vi "HFRR ADV v017 new software.vi"() -> ()   [LabVIEW 2025] (continued)
        n907 = call "IMAGE ANALYSIS.vi"("Enum"=POST_ANALYSIS_ENUM."SHOW UI", "error in"=w1071) -> ("error out"=w1069:errorcluster)  [unwired: 8 in, 1 out]
        n908 = local write "Zoom Factore"(100.0 ("Zoom Factore")) -> ()
      }
    }
    n909 = case shown="True" w760 {
      selector: w760 -> [_ w1048]
      tunnel: w752 -> [w1045 w1053]
      tunnel: [w1045 w1047] -> _
      frame False {
      }
      frame True {
        n910 = Not(x=w1048) -> (.not. x?=w1046:bool)
        n911 = local read "Zoom Factore"() -> (w1051:dbl)
        n912 = local write "OUT"(w1046) -> ()
        n913 = call "IMAGE ANALYSIS.vi"("Enum"=POST_ANALYSIS_ENUM."ZOOM OUT", "error in"=w1053) -> ("error out"=w1047:errorcluster)  [unwired: 8 in, 1 out]
        n914 = Divide(x=w1051, y=1.2) -> (x/y=w1049:dbl)
        n915 = local write "Zoom Factore"(w1049) -> ()
      }
    }
    n916 = case shown="True" w761 {
      selector: w761 -> [_ w1057]
      tunnel: w752 -> [w1054 w1062]
      tunnel: [w1054 w1055] -> _
      frame False {
      }
      frame True {
        n917 = Not(x=w1057) -> (.not. x?=w1056:bool)
        n918 = local read "Zoom Factore"() -> (w1060:dbl)
        n919 = local write "In"(w1056) -> ()
        n920 = call "IMAGE ANALYSIS.vi"("Enum"=POST_ANALYSIS_ENUM."ZOOM IN", "error in"=w1062) -> ("error out"=w1055:errorcluster)  [unwired: 8 in, 1 out]
        n921 = Multiply(x=w1060, y=1.2) -> (x*y=w1058:dbl)
        n922 = local write "Zoom Factore"(w1058) -> ()
      }
    }
    n923 = case shown="True" w757 {
      selector: w757 -> [_ w1029]
      tunnel: w752 -> [w1027 w1031]
      tunnel: [w1027 w1030] -> _
      frame False {
      }
      frame True {
        n924 = Not(x=w1029) -> (.not. x?=w1028:bool)
        n925 = local write "Clear ROI Tool"(w1028) -> ()
        n926 = call "IMAGE ANALYSIS.vi"("Enum"=POST_ANALYSIS_ENUM."CLEAR ROI", "error in"=w1031) -> ("error out"=w1030:errorcluster)  [unwired: 8 in, 1 out]
      }
    }
    n927 = case shown="True" w759 {
      selector: w759 -> [_ w1041]
      tunnel: w752 -> [w1039 w1044]
      tunnel: [w1039 w1042] -> _
      frame False {
      }
      frame True {
        n928 = Not(x=w1041) -> (.not. x?=w1040:bool)
        n929 = local write "line tool"(w1040) -> ()
        n930 = call "IMAGE ANALYSIS.vi"("Enum"=POST_ANALYSIS_ENUM."DRAW LINE", "error in"=w1044) -> ("error out"=w1042:errorcluster)  [unwired: 8 in, 1 out]
      }
    }
    n931 = case shown="True" w758 {
      selector: w758 -> [_ w1035]
      tunnel: w752 -> [w1033 w1037]
      tunnel: [w1033 w1036] -> _
      frame False {
      }
      frame True {
        n932 = Not(x=w1035) -> (.not. x?=w1034:bool)
        n933 = local write "Rectangle Tool"(w1034) -> ()
        n934 = call "IMAGE ANALYSIS.vi"("Enum"=POST_ANALYSIS_ENUM."DRAW REC", "error in"=w1037) -> ("error out"=w1036:errorcluster)  [unwired: 8 in, 1 out]
      }
    }
    n935 = local read "SCAR MEASURMENT"() -> (w745:enum32{"Auto Scar", "Manual Scar"})
    n936 = local read "Fit to Screen Tool"() -> (w754:bool)
    n937 = local read "Resize Tool"() -> (w753:bool)
    n938 = case shown="\"Manual Scar\", Default" w745 {
      frame "Auto Scar" {
        n939 = property on="Cap Live Image" class="Bool (strict)"("BoolText.Text"="Report" ("Boolean Text.Text")) -> ()  [unwired: 2 in, 2 out]
      }
      frame "Manual Scar", Default {
        n940 = property on="Cap Live Image" class="Bool (strict)"("BoolText.Text"="Save Image" ("Boolean Text.Text")) -> ()  [unwired: 2 in, 2 out]
      }
    }
    n941 = local read "ROI Color Tool"() -> (w755:bool)
    n942 = local read "Pan Tool"() -> (w756:bool)
    n943 = case shown="True" w756 {
      selector: w756 -> [_ w1023]
      tunnel: w752 -> [w1021 w1025]
      tunnel: [w1021 w1024] -> _
      frame False {
      }
      frame True {
        n944 = Not(x=w1023) -> (.not. x?=w1022:bool)
        n945 = call "IMAGE ANALYSIS.vi"("Enum"=POST_ANALYSIS_ENUM."PAN", "error in"=w1025) -> ("error out"=w1024:errorcluster)  [unwired: 8 in, 1 out]
        n946 = local write "Pan Tool"(w1022) -> ()
      }
    }
    n947 = case shown="True" w753 {
      selector: w753 -> [_ w1007]
      tunnel: w752 -> [w1002 w1004]
      tunnel: [w1002 w1003] -> _
      frame False {
      }
      frame True {
        n948 = Not(x=w1007) -> (.not. x?=w1006:bool)
        n949 = local write "Resize Tool"(w1006) -> ()
        n950 = call "IMAGE ANALYSIS.vi"("Enum"=POST_ANALYSIS_ENUM."RESIZE MODE", "error in"=w1004) -> ("error out"=w1003:errorcluster)  [unwired: 8 in, 1 out]
      }
    }
    n951 = case shown="True" w754 {
      selector: w754 -> [_ w1012]
      tunnel: [w1008 w1013] -> _
      tunnel: w752 -> [w1008 w1011]
      frame False {
      }
      frame True {
        n952 = Not(x=w1012) -> (.not. x?=w1010:bool)
        n953 = local write "Zoom Factore"(100.0 ("Zoom Factore")) -> ()
        n954 = local write "Fit to Screen Tool"(w1010) -> ()
        n955 = call "IMAGE ANALYSIS.vi"("Enum"=POST_ANALYSIS_ENUM."FIT", "error in"=w1011) -> ("error out"=w1013:errorcluster)  [unwired: 8 in, 1 out]
      }
    }
    n956 = case shown="True" w755 {
      selector: w755 -> [_ w1018]
      tunnel: [w1015 w1019] -> _
      tunnel: w752 -> [w1015 w1016]
      frame False {
      }
      frame True {
        n957 = Not(x=w1018) -> (.not. x?=w1017:bool)
        n958 = local write "ROI Color Tool"(w1017) -> ()
        n959 = call "IMAGE ANALYSIS.vi"("Enum"=POST_ANALYSIS_ENUM."SET ROI COLOR", "error in"=w1016) -> ("error out"=w1019:errorcluster)  [unwired: 8 in, 1 out]
      }
    }
    n960 = local read "Quit"() -> (w769:bool)
  }
  n961 = while {
    stop <- w1103 stop-if-true
    n962 = local read "Image Path"() -> (w1106:path)
    n963 = local read "Print 3"() -> (w1109:bool)
    n964 = Equal?(x=w1106, y=path "") -> (x = y?=w1105:bool)
    n965 = Not(x=w1105) -> (.not. x?=w1104:bool)
    n966 = property on="Print 3" class="Bool (strict)"("Visible"=w1104) -> ()  [unwired: 2 in, 2 out]
    n967 = case shown="True" w1109 {
      frame False {
        n968 = local write "Rd"(TRUE ("Boolean 7")) -> ()
      }
      frame True {
        n969 = flat-sequence {
          tunnel: [w1149] -> w1117
          tunnel: [w1136] -> w1115
          tunnel: [w1146] -> w1111
          tunnel: w1117 -> [w1158]
          tunnel: [w1158] -> w1116
          tunnel: w1115 -> [w1157]
          tunnel: [w1157] -> w1114
          tunnel: [w1155] -> w1113
          tunnel: [w1154] -> w1112
          tunnel: w1111 -> [w1154]
          tunnel: w1116 -> [w1160]
          tunnel: w1114 -> [w1161]
          tunnel: w1113 -> [_]
          tunnel: w1112 -> [w1159]
          frame #0 {
            n970 = case shown="True" "Rd" {
              frame False {
              }
              frame True {
                n971 = while {
                  tunnel: "abcdefABCDEF" ("string 2") -> [w1128]
                  shift-right: [w1126] -> w1120
                  shift-left: "" -> [w1125]
                  i -> [w1135]
                  stop <- w1134 stop-if-true
                  n972 = Random Number (0-1)() -> (number: 0 to 1=w1129:dbl)
                  n973 = Multiply(x=w1129, y=62.0) -> (x*y=w1131:dbl)
                  n974 = Decrement(x="Length 2") -> (x-1=w1124:i16)
                  n975 = To Word Integer(number=w1131) -> (16bit integer=w1132:i16)
                  n976 = String Subset(string=w1128, offset (0)=w1132, length (rest)=1 ("length (rest)")) -> (substring=w1127:string)
                  n977 = Greater Or Equal?(x=w1135, y=w1124) -> (x >= y?=w1134:bool)
                  n978 = Concatenate Strings(w1127, w1125) -> (w1126:string)
                }
                "String 10" <- w1120
                n979 = local write "Rd"(FALSE ("Boolean 7")) -> ()
              }
            }
          }
          frame #1 {
            w1147 = "_resized.jpg" ("command line")
            (unwired) ".jpg -resize 320x240 " ("string")
            (unwired) "Choose an Image File" ("prompt")
            # "-resize 1798x425"
            n980 = local read "Image Path"() -> (w1141:path)
            n981 = Strip Path(path=w1141) -> (stripped path=w1136:path, name=w1137:string)
            n982 = Match Pattern(string=w1137, regular expression=".jpg") -> (before substring=→"before substring 2":string, after substring=→"after substring":string)  [unwired: 1 in, 2 out]
            n983 = Match Pattern(string=w1137, regular expression="\\") -> (before substring=w1143:string)  [unwired: 1 in, 3 out]
            n984 = Match Pattern(string=w1143, regular expression=".jpg") -> (before substring=w1142:string)  [unwired: 1 in, 3 out]
            n985 = Concatenate Strings("cmd /c convert " ("string"), w1142, ".jpg -resize 320x240  " ("command line"), w1142, w1147) -> (w1150:string)
            n986 = call <vilib>:"System Exec.vi"("run minimized? (F)"=TRUE, "wait until completion? (T)"=TRUE, "working directory"=w1136, "command line"=w1150) -> ("error out"=w1149:errorcluster)  [unwired: 4 in, 3 out]
            "error out 2" <- w1149
            n987 = Concatenate Strings(w1142, w1147) -> (w1146:string)
          }
          frame #2 {
            n988 = Wait (ms)(milliseconds to wait=u32 2000 ("millisecond timer value")) -> (millisecond timer value=w1155:u32)
          }
          frame #3 {
            n989 = case shown="No Error" w1160 {
              tunnel: w1161 -> [w1164 _]
              tunnel: w1159 -> [w1162 _]
              frame No Error {
                (unwired) ".jpg" ("string")
                n990 = Path To String(path=w1164) -> (string=w1168:string)
                n991 = Concatenate Strings(w1168, "\\" ("string"), w1162) -> (w1167:string)
                n992 = String To Path(string=w1167) -> (path=w1166:path)
                n993 = call <vilib>:"Read JPEG File.vi"("path to JPEG file"=w1166) -> ("image data"=w1170:T16)  [unwired: 8 in, 2 out]
                "image data" <- w1170
                n994 = local write "Print 3"(FALSE ("Print 2")) -> ()
                n995 = call <vilib>:"Draw Flattened Pixmap.vi"("image data"=w1170) -> ("new picture"=→"new picture":picture)  [unwired: 8 in]
              }
              frame Error {
              }
            }
          }
        }
      }
    }
    n996 = Wait (ms)(milliseconds to wait=u32 20 ("millisecond timer value")) -> ()  [unwired: 1 out]
    n997 = local read "Quit"() -> (w1103:bool)
  }
  n998 = while {
    tunnel: w34 -> [_]
    tunnel: w18 -> [_]
    stop <- w1201 stop-if-true
    # "New Adv Logics"
    n999 = local read "Main Tab"() -> (w1181:T2)
    n1000 = local read "Main Tab"() -> (w1199:T2)
    n1001 = local read "Sign In"() -> (w1198:bool)
    n1002 = case shown="\"Adv Scar\"" w1181 {
      frame "HOME", Default {
        n1003 = local read "LIVE FEED MIN TEMP"() -> (w1334:bool)
        n1004 = local write "LIVE FEED MAX TEMP"(TRUE ("LIVE FEED MAX TEMP")) -> ()
        n1005 = local read "CAMERA ROI MIN TEMP"() -> (w1332:bool)
        n1006 = case shown="True" w1334 {
          selector: w1334 -> [_ w1341]
          frame False {
          }
          frame True {
            n1007 = Not(x=w1341) -> (.not. x?=w1340:bool)
            n1008 = local write "LIVE FEED MIN TEMP"(w1340) -> ()
            n1009 = call "CAMERA LIVE FEED FGV.vi"("Enum - Menu"=CAMERA_LIVE_FEED_ENUM."CAMERA MINIMIZE") -> ()  [unwired: 9 in, 2 out]
          }
        }
        n1010 = case shown="True" w1332 {
          selector: w1332 -> [_ w1338]
          frame False {
          }
          frame True {
            n1011 = Not(x=w1338) -> (.not. x?=w1337:bool)
            n1012 = local write "CAMERA ROI MIN TEMP"(w1337) -> ()
            n1013 = call "IMAGE ANALYSIS.vi"("Enum"=POST_ANALYSIS_ENUM."MINIMIZE UI") -> ()  [unwired: 9 in, 2 out]
          }
        }
        n1014 = local write "CAMERA ROI MAX TEMP"(TRUE ("CAMERA ROI MAX TEMP")) -> ()
      }
      frame "Test Setup" {
        n1015 = local read "LIVE FEED MIN TEMP"() -> (w1344:bool)
        n1016 = local read "CAMERA ROI MIN TEMP"() -> (w1342:bool)
        n1017 = local write "LIVE FEED MAX TEMP"(TRUE ("LIVE FEED MAX TEMP")) -> ()
        n1018 = case shown="True" w1344 {
          selector: w1344 -> [_ w1351]
          frame False {
          }
          frame True {
            n1019 = Not(x=w1351) -> (.not. x?=w1350:bool)
            n1020 = local write "LIVE FEED MIN TEMP"(w1350) -> ()
            n1021 = call "CAMERA LIVE FEED FGV.vi"("Enum - Menu"=CAMERA_LIVE_FEED_ENUM."CAMERA MINIMIZE") -> ()  [unwired: 9 in, 2 out]
          }
        }
        n1022 = case shown="True" w1342 {
          selector: w1342 -> [_ w1348]
          frame False {
          }
          frame True {
            n1023 = Not(x=w1348) -> (.not. x?=w1347:bool)
            n1024 = local write "CAMERA ROI MIN TEMP"(w1347) -> ()
            n1025 = call "IMAGE ANALYSIS.vi"("Enum"=POST_ANALYSIS_ENUM."MINIMIZE UI") -> ()  [unwired: 9 in, 2 out]
          }
        }
        n1026 = local write "CAMERA ROI MAX TEMP"(TRUE ("CAMERA ROI MAX TEMP")) -> ()
      }
      frame "Acquire" {
        n1027 = local read "LIVE FEED MIN TEMP"() -> (w1354:bool)
        n1028 = local write "LIVE FEED MAX TEMP"(TRUE ("LIVE FEED MAX TEMP")) -> ()
        n1029 = local read "CAMERA ROI MIN TEMP"() -> (w1352:bool)
        n1030 = case shown="True" w1354 {
          selector: w1354 -> [_ w1361]
          frame False {
          }
          frame True {
            n1031 = Not(x=w1361) -> (.not. x?=w1360:bool)
            n1032 = local write "LIVE FEED MIN TEMP"(w1360) -> ()
            n1033 = call "CAMERA LIVE FEED FGV.vi"("Enum - Menu"=CAMERA_LIVE_FEED_ENUM."CAMERA MINIMIZE") -> ()  [unwired: 9 in, 2 out]
          }
        }
        n1034 = case shown="True" w1352 {
          selector: w1352 -> [_ w1358]
          frame False {
          }
          frame True {
            n1035 = Not(x=w1358) -> (.not. x?=w1357:bool)
            n1036 = local write "CAMERA ROI MIN TEMP"(w1357) -> ()
            n1037 = call "IMAGE ANALYSIS.vi"("Enum"=POST_ANALYSIS_ENUM."MINIMIZE UI") -> ()  [unwired: 9 in, 2 out]
          }
        }
        n1038 = local write "CAMERA ROI MAX TEMP"(TRUE ("CAMERA ROI MAX TEMP")) -> ()
      }
      frame "Adv Scar" {
        n1039 = local read "CAMERA ROI MIN TEMP"() -> (w1362:bool)
        n1040 = case shown="True" "LIVE FEED MAX TEMP" {
          selector: "LIVE FEED MAX TEMP" -> [_ w1383]
          frame False {
          }
          frame True {
            n1041 = Not(x=w1383) -> (.not. x?=w1382:bool)
            n1042 = local write "LIVE FEED MAX TEMP"(w1382) -> ()
            n1043 = call "CAMERA LIVE FEED FGV.vi"("Enum - Menu"=CAMERA_LIVE_FEED_ENUM."CAMERA RESTORE") -> ("error out"=w1373:errorcluster)  [unwired: 9 in, 1 out]
            n1044 = Type Cast(type=30, x=0) -> (*(type *) &x=w1377:i32)
            n1045 = Add(x=w1377, y=48) -> (x+y=w1378:i32)
            n1046 = call "CAMERA LIVE FEED FGV.vi"("Enum - Menu"=CAMERA_LIVE_FEED_ENUM."CAMERA MODE SET", "error in (no error)"=w1373, "CAMERA MODE"=w1378) -> ("error out"=w1370:errorcluster)  [unwired: 7 in, 1 out]
            n1047 = call "CAMERA LIVE FEED FGV.vi"("Enum - Menu"=CAMERA_LIVE_FEED_ENUM."CAMERA GRAY", "error in (no error)"=w1370) -> ("error out"=w1369:errorcluster)  [unwired: 8 in, 1 out]
            n1048 = call "LIST FILE NAMES.vi"("error in (no error)"=w1369) -> ("error out"=w1379:errorcluster, "filenames"=w1380:string[])  [unwired: 9 in]
            n1049 = property on="FILE 3" class="CmbBox"(error in=w1379, "Strings[]"=w1380) -> ()  [unwired: 1 in, 2 out]
          }
        }
        n1050 = case shown="True" w1362 {
          selector: w1362 -> [_ w1368]
          frame False {
          }
          frame True {
            n1051 = Not(x=w1368) -> (.not. x?=w1367:bool)
            n1052 = local write "CAMERA ROI MIN TEMP"(w1367) -> ()
            n1053 = call "IMAGE ANALYSIS.vi"("Enum"=POST_ANALYSIS_ENUM."MINIMIZE UI") -> ()  [unwired: 9 in, 2 out]
          }
        }
        n1054 = local write "CAMERA ROI MAX TEMP"(TRUE ("CAMERA ROI MAX TEMP")) -> ()
        "LIVE FEED MIN TEMP" <- TRUE ("LIVE FEED MIN TEMP")
      }
      frame "Adv Scar Report" {
        n1055 = local read "CAMERA ROI MAX TEMP"() -> (w1384:bool)
        n1056 = local read "LIVE FEED MIN TEMP"() -> (w1386:bool)
        n1057 = local write "LIVE FEED MAX TEMP"(TRUE ("LIVE FEED MAX TEMP")) -> ()
        n1058 = case shown="True" w1386 {
          selector: w1386 -> [_ w1395]
          frame False {
          }
          frame True {
            n1059 = Not(x=w1395) -> (.not. x?=w1394:bool)
            n1060 = local write "LIVE FEED MIN TEMP"(w1394) -> ()
            n1061 = call "CAMERA LIVE FEED FGV.vi"("Enum - Menu"=CAMERA_LIVE_FEED_ENUM."CAMERA MINIMIZE") -> ()  [unwired: 9 in, 2 out]
          }
        }
        n1062 = case shown="True" w1384 {
          selector: w1384 -> [_ w1392]
          frame False {
          }
          frame True {
            n1063 = Not(x=w1392) -> (.not. x?=w1390:bool)
            n1064 = local write "CAMERA ROI MAX TEMP"(w1390) -> ()
            n1065 = call "IMAGE ANALYSIS.vi"("Enum"=POST_ANALYSIS_ENUM."SHOW UI") -> ("error out"=w1389:errorcluster)  [unwired: 9 in, 1 out]
            n1066 = call "LIST FILE NAMES.vi"("error in (no error)"=w1389) -> ("filenames"=w1388:string[])  [unwired: 9 in, 1 out]
            n1067 = property on="Test File List :" class="CmbBox"("Strings[]"=w1388) -> ()  [unwired: 2 in, 2 out]
          }
        }
        n1068 = local write "CAMERA ROI MIN TEMP"(TRUE ("CAMERA ROI MIN TEMP")) -> ()
      }
      frame "Compare Files" {
        n1069 = local read "LIVE FEED MIN TEMP"() -> (w1398:bool)
        n1070 = local write "LIVE FEED MAX TEMP"(TRUE ("LIVE FEED MAX TEMP")) -> ()
        n1071 = local read "CAMERA ROI MIN TEMP"() -> (w1396:bool)
        n1072 = case shown="True" w1398 {
          selector: w1398 -> [_ w1405]
          frame False {
          }
          frame True {
            n1073 = Not(x=w1405) -> (.not. x?=w1404:bool)
            n1074 = local write "LIVE FEED MIN TEMP"(w1404) -> ()
            n1075 = call "CAMERA LIVE FEED FGV.vi"("Enum - Menu"=CAMERA_LIVE_FEED_ENUM."CAMERA MINIMIZE") -> ()  [unwired: 9 in, 2 out]
          }
        }
        n1076 = case shown="True" w1396 {
          selector: w1396 -> [_ w1402]
          frame False {
          }
          frame True {
            n1077 = Not(x=w1402) -> (.not. x?=w1401:bool)
            n1078 = local write "CAMERA ROI MIN TEMP"(w1401) -> ()
            n1079 = call "IMAGE ANALYSIS.vi"("Enum"=POST_ANALYSIS_ENUM."MINIMIZE UI") -> ()  [unwired: 9 in, 2 out]
          }
        }
        n1080 = local write "CAMERA ROI MAX TEMP"(TRUE ("CAMERA ROI MAX TEMP")) -> ()
      }
      frame "About" {
        n1081 = local read "LIVE FEED MIN TEMP"() -> (w1408:bool)
        n1082 = local write "LIVE FEED MAX TEMP"(TRUE ("LIVE FEED MAX TEMP")) -> ()
        n1083 = local read "CAMERA ROI MIN TEMP"() -> (w1407:bool)
        n1084 = case shown="True" w1408 {
          selector: w1408 -> [_ w1415]
          frame False {
          }
          frame True {
            n1085 = Not(x=w1415) -> (.not. x?=w1414:bool)
            n1086 = local write "LIVE FEED MIN TEMP"(w1414) -> ()
            n1087 = call "CAMERA LIVE FEED FGV.vi"("Enum - Menu"=CAMERA_LIVE_FEED_ENUM."CAMERA MINIMIZE") -> ()  [unwired: 9 in, 2 out]
          }
        }
        n1088 = case shown="True" w1407 {
          selector: w1407 -> [_ w1412]
          frame False {
          }
          frame True {
            n1089 = Not(x=w1412) -> (.not. x?=w1411:bool)
            n1090 = local write "CAMERA ROI MIN TEMP"(w1411) -> ()
            n1091 = call "IMAGE ANALYSIS.vi"("Enum"=POST_ANALYSIS_ENUM."MINIMIZE UI") -> ()  [unwired: 9 in, 2 out]
          }
        }
        n1092 = local write "CAMERA ROI MAX TEMP"(TRUE ("CAMERA ROI MIN TEMP")) -> ()
      }
      frame "Advance" {
        n1093 = local read "LIVE FEED MIN TEMP"() -> (w1418:bool)
        n1094 = local write "LIVE FEED MAX TEMP"(TRUE ("LIVE FEED MAX TEMP")) -> ()
        n1095 = local read "CAMERA ROI MIN TEMP"() -> (w1416:bool)
        n1096 = case shown="True" w1418 {
          selector: w1418 -> [_ w1425]
          frame False {
          }
          frame True {
            n1097 = Not(x=w1425) -> (.not. x?=w1424:bool)
            n1098 = local write "LIVE FEED MIN TEMP"(w1424) -> ()
            n1099 = call "CAMERA LIVE FEED FGV.vi"("Enum - Menu"=CAMERA_LIVE_FEED_ENUM."CAMERA MINIMIZE") -> ()  [unwired: 9 in, 2 out]
          }
        }
        n1100 = local write "CAMERA ROI MAX TEMP"(TRUE ("CAMERA ROI MAX TEMP")) -> ()
        n1101 = case shown="True" w1416 {
          selector: w1416 -> [_ w1422]
          frame False {
          }
          frame True {
            n1102 = Not(x=w1422) -> (.not. x?=w1421:bool)
            n1103 = local write "CAMERA ROI MIN TEMP"(w1421) -> ()
            n1104 = call "IMAGE ANALYSIS.vi"("Enum"=POST_ANALYSIS_ENUM."MINIMIZE UI") -> ()  [unwired: 9 in, 2 out]
          }
        }
      }
      frame "Mooha" {
        n1105 = local read "LIVE FEED MIN TEMP"() -> (w1428:bool)
        n1106 = local write "LIVE FEED MAX TEMP"(TRUE ("LIVE FEED MAX TEMP")) -> ()
        n1107 = local read "CAMERA ROI MIN TEMP"() -> (w1426:bool)
        n1108 = case shown="True" w1428 {
          selector: w1428 -> [_ w1435]
          frame False {
          }
          frame True {
            n1109 = Not(x=w1435) -> (.not. x?=w1434:bool)
            n1110 = local write "LIVE FEED MIN TEMP"(w1434) -> ()
            n1111 = call "CAMERA LIVE FEED FGV.vi"("Enum - Menu"=CAMERA_LIVE_FEED_ENUM."CAMERA MINIMIZE") -> ()  [unwired: 9 in, 2 out]
          }
        }
        n1112 = local write "CAMERA ROI MAX TEMP"(TRUE ("CAMERA ROI MAX TEMP")) -> ()
        n1113 = case shown="True" w1426 {
          selector: w1426 -> [_ w1432]
          frame False {
          }
          frame True {
            n1114 = Not(x=w1432) -> (.not. x?=w1431:bool)
            n1115 = local write "CAMERA ROI MIN TEMP"(w1431) -> ()
            n1116 = call "IMAGE ANALYSIS.vi"("Enum"=POST_ANALYSIS_ENUM."MINIMIZE UI") -> ()  [unwired: 9 in, 2 out]
          }
        }
      }
    }
    n1117 = local read "Auto Start Test"() -> (w1172:bool)
    n1118 = case shown="True" "sign in temp" {
      frame False {
      }
      frame True {
        w1208 = 1 ("y")
        n1119 = local read "USERNAME"() -> (w1214:string)
        n1120 = local read "USER ID"() -> (w1211:string)
        n1121 = call <vilib>:"Trim Whitespace.vi"("string"=w1214) -> ("trimmed string"=w1213:string)  [unwired: 1 in]
        n1122 = call <vilib>:"Trim Whitespace.vi"("string"=w1211) -> ("trimmed string"=w1212:string)  [unwired: 1 in]
        n1123 = String Length(string=w1213) -> (length=w1210:i32)
        n1124 = String Length(string=w1212) -> (length=w1209:i32)
        n1125 = Greater?(x=w1210, y=w1208) -> (0:w1207:bool)
        n1126 = Greater?(x=w1209, y=w1208) -> (0:w1206:bool)
        n1127 = And(x=w1207, y=w1206) -> (x .and. y?=w1205:bool)
        n1128 = case shown="True" w1205 {
          frame False {
            n1129 = property on="Sign In" class="Bool (strict)"("DisabledEnum"=T19."Disabled" ("Disabled")) -> ()  [unwired: 2 in, 2 out]
          }
          frame True {
            n1130 = property on="Sign In" class="Bool (strict)"("DisabledEnum"=T19."Enabled" ("Disabled")) -> ()  [unwired: 2 in, 2 out]
          }
        }
      }
    }
    n1131 = local read "Air Temperature"() -> (w1189:bool)
    n1132 = local read "Coefficient Of Friction"() -> (w1190:bool)
    n1133 = case shown="False" w1172 {
      frame False {
        n1134 = local read "Auto stop temp"() -> (w1202:bool)
        n1135 = case shown="True" w1202 {
          frame False {
          }
          frame True {
            n1136 = local write "Auto Start Temp"(FALSE ("Auto Start Temp")) -> ()
          }
        }
      }
      frame True {
        "Auto stop temp" <- TRUE ("Auto stop temp")
      }
    }
    n1137 = local read "Humidity"() -> (w1188:bool)
    n1138 = case shown="\"HOME\"" w1199 {
      frame "HOME" {
        n1139 = local write "main tab sub"(enum32{"Page 1", "Page 2"}."Page 1" ("main tab sub")) -> ()
      }
      frame Default {
        n1140 = local write "main tab sub"(enum32{"Page 1", "Page 2"}."Page 2" ("main tab sub")) -> ()
      }
    }
    n1141 = case shown="True" w1198 {
      selector: w1198 -> [_ w1549]
      frame False {
      }
      frame True {
        n1142 = Not(x=w1549) -> (.not. x?=w1548:bool)
        n1143 = local write "Sign In"(w1548) -> ()
        n1144 = local write "Main Dashboard Buttons"(T24."Test Setup" ("Main Dashboard Buttons")) -> ()
      }
    }
    n1145 = case shown="\"Numeric Display\", Default" "Num/Graph" {
      frame "Numeric Display", Default {
        n1146 = property on="Single/Multiple" class="RadioBtnsControl (strict)"("Visible"=FALSE) -> ()  [unwired: 2 in, 2 out]
        n1147 = property on="Single - Graph" class="Ring (strict)"("Visible"=FALSE) -> ()  [unwired: 2 in, 2 out]
        n1148 = local write "Main Tab Display"(T4."Dashboard 1" ("Main Tab Display")) -> ()
      }
      frame "Graph Display" {
        n1149 = property on="Single/Multiple" class="RadioBtnsControl (strict)"("Visible"=TRUE) -> ()  [unwired: 2 in, 2 out]
        n1150 = case shown="\"Multiple\"" "Single/Multiple" {
          frame "Single ", Default {
            n1151 = property on="Single - Graph" class="Ring (strict)"("Visible"=TRUE) -> ()  [unwired: 2 in, 2 out]
            n1152 = local write "Main Tab Display"(T4."Dashboard 3" ("Main Tab Display")) -> ()
          }
          frame "Multiple" {
            n1153 = property on="Single - Graph" class="Ring (strict)"("Visible"=FALSE) -> ()  [unwired: 2 in, 2 out]
            n1154 = local write "Main Tab Display"(T4."Dashboard 2" ("Main Tab Display")) -> ()
          }
        }
      }
    }
    n1155 = local read "Stroke"() -> (w1187:bool)
    n1156 = local read "USERNAME"() -> (w1193:string)
    n1157 = local read "USER ID"() -> (w1192:string)
    n1158 = case shown="True" w1190 {
      selector: w1190 -> [_ w1475]
      frame False {
      }
      frame True {
        n1159 = Not(x=w1475) -> (.not. x?=w1474:bool)
        n1160 = local write "Coefficient Of Friction"(w1474) -> ()
        n1161 = local write "Tab Control 2"(T6."Coefficient Of Friction" ("Tab Control 2")) -> ()
      }
    }
    n1162 = case shown="True" w1189 {
      selector: w1189 -> [_ w1472]
      frame False {
      }
      frame True {
        n1163 = Not(x=w1472) -> (.not. x?=w1470:bool)
        n1164 = local write "Air Temperature"(w1470) -> ()
        n1165 = local write "Tab Control 2"(T6."Air Temperature" ("Tab Control 2")) -> ()
      }
    }
    n1166 = local write "Operator ID"(w1192) -> ()
    n1167 = case shown="True" w1187 {
      selector: w1187 -> [_ w1466]
      frame False {
      }
      frame True {
        n1168 = Not(x=w1466) -> (.not. x?=w1464:bool)
        n1169 = local write "Stroke"(w1464) -> ()
        n1170 = local write "Tab Control 2"(T6."Stroke" ("Tab Control 2")) -> ()
      }
    }
    n1171 = local write "tested by"(w1193) -> ()
    n1172 = case shown="True" w1188 {
      selector: w1188 -> [_ w1469]
      frame False {
      }
      frame True {
        n1173 = Not(x=w1469) -> (.not. x?=w1467:bool)
        n1174 = local write "Humidity"(w1467) -> ()
        n1175 = local write "Tab Control 2"(T6."Humidity" ("Tab Control 2")) -> ()
      }
    }
    n1176 = case shown="\"Calibration\"" "Main Dashboard Buttons" {
      tunnel: [T2."HOME" ("Main Tab") T2."Test Setup" ("Main Tab") T2."Acquire" ("Main Tab") T2."Adv Scar" ("Main Tab") T2."Adv Scar Report" ("Main Tab") T2."Compare Files" ("Main Tab") T2."Calibration" ("Main Tab") T2."About" ("Main Tab") T2."Advance" ("Main Tab")] -> w1171
      frame "Home", Default {
      }
      frame "Test Setup" {
      }
      frame "Dashboard" {
      }
      frame "Imaging" {
      }
      frame "Report" {
      }
      frame "Analysis" {
      }
      frame "Calibration" {
      }
      frame "About" {
      }
      frame "Advance" {
      }
    }
    n1177 = Wait (ms)(milliseconds to wait=u32 100) -> ()  [unwired: 1 out]
    n1178 = local read "Main Tab Display"() -> (w1191:T4)
    n1179 = local write "Main Tab"(w1171) -> ()
    n1180 = case shown="\"Dashboard 3\"" w1191 {
      frame "Dashboard 1", Default {
        n1181 = property on="Reset Graph" class="Bool (strict)"("Visible"=FALSE) -> ()  [unwired: 2 in, 2 out]
      }
      frame "Dashboard 2" {
        n1182 = property on="Reset Graph" class="Bool (strict)"("Visible"=TRUE) -> ()  [unwired: 2 in, 2 out]
      }
      frame "Dashboard 3" {
        n1183 = property on="Reset Graph" class="Bool (strict)"("Visible"=TRUE) -> ()  [unwired: 2 in, 2 out]
      }
    }
    n1184 = local read "SCAR MEASURMENT"() -> (w1179:enum32{"Auto Scar", "Manual Scar"})
    n1185 = local read "Humidity"() -> (w1194:bool)
    n1186 = local read "Cap Live Image"() -> (w1176:bool)
    n1187 = local read "Sample Temperature"() -> (w1186:bool)
    n1188 = local read "Air Temp vs Humidity"() -> (w1184:bool)
    n1189 = local read "Frequency"() -> (w1185:bool)
    n1190 = case shown="True" w1194 {
      frame False {
        n1191 = local write "Humidity On Command"(TRUE ("Humidity On Command")) -> ()
        n1192 = case shown="True" "Humidity Off Command" {
          selector: "Humidity Off Command" -> [_ w1482]
          frame False {
          }
          frame True {
            n1193 = stacked-sequence {
              frame #0 {
                n1194 = local read "WriteHumidity"() -> (w1484:string[])
                n1195 = Insert Into Array(array=w1484, new element="R;1" ("new element/subarray")) -> (w1485:string[])  [unwired: 1 in]
                n1196 = local write "WriteHumidity"(w1485) -> ()
              }
              frame #1 {
                n1197 = Wait (ms)(milliseconds to wait=u32 2000) -> ()  [unwired: 1 out]
              }
              frame #2 {
                n1198 = local read "EVENT LOG"() -> (w1491:string)
                n1199 = local read "WriteHumidity"() -> (w1488:string[])
                n1200 = call "Event Log.vi"("Content"="Humidity Control Off" ("string"), "EVENT LOG"=w1491) -> ("EVENT LOG"=w1492:string)  [unwired: 8 in, 1 out]
                n1201 = local write "EVENT LOG"(w1492) -> ()
                n1202 = Insert Into Array(array=w1488, new element="R;1" ("new element/subarray")) -> (w1489:string[])  [unwired: 1 in]
                n1203 = local write "WriteHumidity"(w1489) -> ()
              }
            }
            n1204 = Not(x=w1482) -> (.not. x?=w1481:bool)
            n1205 = local write "Humidity Off Command"(w1481) -> ()
          }
        }
      }
      frame True {
        n1206 = local write "Humidity Off Command"(TRUE ("Humidity Off Command")) -> ()
        n1207 = case shown="True" "Humidity On Command" {
          selector: "Humidity On Command" -> [_ w1496]
          frame False {
          }
          frame True {
            n1208 = stacked-sequence {
              frame #0 {
                n1209 = local read "Set Rh"() -> (w1502:dbl)
                n1210 = Number To Fractional String(number=w1502, precision (6)=i16 2) -> (F-format string=w1503:string)  [unwired: 2 in]
                n1211 = local read "WriteHumidity"() -> (w1500:string[])
                n1212 = Concatenate Strings("M;" ("new element/subarray"), w1503) -> (w1501:string)
                n1213 = Insert Into Array(array=w1500, new element=w1501) -> (w1499:string[])  [unwired: 1 in]
                n1214 = local write "WriteHumidity"(w1499) -> ()
              }
              frame #1 {
                n1215 = Wait (ms)(milliseconds to wait=u32 2000) -> ()  [unwired: 1 out]
              }
              frame #2 {
                n1216 = local read "Set Rh"() -> (w1510:dbl)
                n1217 = Number To Fractional String(number=w1510, precision (6)=i16 2) -> (F-format string=w1511:string)  [unwired: 2 in]
                n1218 = local read "WriteHumidity"() -> (w1508:string[])
                n1219 = Concatenate Strings("M;" ("new element/subarray"), w1511) -> (w1509:string)
                n1220 = Insert Into Array(array=w1508, new element=w1509) -> (w1507:string[])  [unwired: 1 in]
                n1221 = local write "WriteHumidity"(w1507) -> ()
              }
              frame #3 {
                n1222 = Wait (ms)(milliseconds to wait=u32 1500) -> ()  [unwired: 1 out]
              }
              frame #4 {
                (unwired) "% RH" ("string")
                (unwired) i16 2 ("precision (6)")
                (unwired) "M;" ("new element/subarray")
                n1223 = local read "Set Rh"() -> (w1518:dbl)
                n1224 = Number To Fractional String(number=w1518, precision (6)=i16 2) -> (F-format string=w1515:string)  [unwired: 2 in]
                n1225 = local read "WriteHumidity"() -> (w1520:string[])
                n1226 = Concatenate Strings("M;" ("new element/subarray"), w1515) -> (w1519:string)
                n1227 = Concatenate Strings("Humidity Set to : " ("string"), w1515, "% RH" ("string")) -> (w1513:string)
                n1228 = Insert Into Array(array=w1520, new element=w1519) -> (w1521:string[])  [unwired: 1 in]
                n1229 = disable-structure shown="Enabled" {
                  frame Enabled {
                    n1230 = local read "EVENT LOG"() -> (w1524:string)
                    n1231 = call "Event Log.vi"("Content"="Humidity Control On", "EVENT LOG"=w1524) -> ("EVENT LOG"=w1525:string)  [unwired: 8 in, 1 out]
                    n1232 = local write "EVENT LOG"(w1525) -> ()
                  }
                  frame Disabled {
                  }
                }
                n1233 = disable-structure shown="Enabled" {
                  disable-tunnel: w1513 -> [_ _]
                  frame Enabled {
                    n1234 = local read "EVENT LOG"() -> (w1527:string)
                    n1235 = call "Event Log.vi"("Content"="Humidity Control On", "EVENT LOG"=w1527) -> ("EVENT LOG"=w1528:string)  [unwired: 8 in, 1 out]
                    n1236 = local write "EVENT LOG"(w1528) -> ()
                  }
                  frame Disabled {
                  }
                }
                n1237 = local write "WriteHumidity"(w1521) -> ()
              }
            }
            n1238 = Not(x=w1496) -> (.not. x?=w1495:bool)
            n1239 = local write "Humidity On Command"(w1495) -> ()
          }
        }
      }
    }
    n1240 = Equal?(x=w1179, y=enum32{"Auto Scar", "Manual Scar"}."Auto Scar" ("SCAR MEASURMENT")) -> (x = y?=w1175:bool)
    n1241 = local read "TEST STANDARD"() -> (w1182:T3)
    n1242 = And(x=w1176, y=w1175) -> (x .and. y?=w1177:bool)
    n1243 = case shown="True" w1177 {
      selector: w1177 -> [_ w1281]
      tunnel: errorcluster {"status"=FALSE, "code"=0, "source"=""} ("error in (no error) 3") -> [_ w1282]
      frame False {
      }
      frame True {
        n1244 = stacked-sequence {
          tunnel: w1282 -> [_ _ _ _ _ _ _ w1330]
          tunnel: w1281 -> [_ _ _ _ _ w1311 _ _]
          frame #0 {
            n1245 = call "CAMERA LIVE FEED FGV.vi"("Enum - Menu"=CAMERA_LIVE_FEED_ENUM."CAMERA MINIMIZE") -> ()  [unwired: 9 in, 2 out]
          }
          frame #1 {
            n1246 = property on="Auto Scar Check  2" class="Clust (strict)"("Visible"=TRUE) -> ()  [unwired: 2 in, 2 out]
          }
          frame #2 {
            n1247 = String To Path(string="C:\\LAB-IQ\\Image Calibrate v01.dcf") -> (path=w1287:path)
            n1248 = Open/Create/Replace File ("Open File")(file path (use dialog)=w1287) -> (refnum out=w1288:refnum<file>)  [unwired: 5 in, 2 out]
            n1249 = for {
              N: 4 -> [_]
              tunnel: w1288 -> [w1294]
              i -> [w1290]
              n1250 = Read from Text File ("Read File")(file (use dialog)=w1294) -> (text=w1295:string)  [unwired: 3 in, 3 out]
              n1251 = String Subset(string=w1295, offset (0)=6, length (rest)=10 ("length (rest)")) -> (substring=w1291:string)
              n1252 = Fract/Exp String To Number(string=w1291) -> (number=w1289:dbl)  [unwired: 3 in, 1 out]
              n1253 = case shown="0" w1290 {
                tunnel: w1289 -> [w1296 w1297 _ w1298 _]
                frame 0 {
                  "5x Gain" <- w1296
                }
                frame 1 {
                  "10x Gain" <- w1297
                }
                frame 2 {
                }
                frame 3 {
                  "100x gain" <- w1298
                }
                frame 4, Default {
                }
              }
            }
          }
          frame #3 {
            n1254 = local read "FILE 3"() -> (w1304:string)
            n1255 = call <vilib>:"Trim Whitespace.vi"("string"="C:\\LAB-IQ\\images\\") -> ("trimmed string"=w1306:string)  [unwired: 1 in]
            n1256 = String To Path(string=w1306) -> (path=w1305:path)
            n1257 = Concatenate Strings(w1304, ".png" ("string")) -> (w1303:string)
            n1258 = Build Path(base path=w1305, name or relative path=w1303) -> (appended path=w1301:path)
            "Image path" <- w1301
            n1259 = Path To String(path=w1301) -> (string=w1300:string)
            n1260 = call "CAMERA LIVE FEED FGV.vi"("Enum - Menu"=CAMERA_LIVE_FEED_ENUM."CAMERA SAVE", "Image Path"=w1300) -> ()  [unwired: 8 in, 2 out]
          }
          frame #4 {
            n1261 = One Button Dialog(message="Image saved successfully") -> ()  [unwired: 1 in, 1 out]
          }
          frame #5 {
            n1262 = local read "TEST STANDARD"() -> (w1310:T3)
            n1263 = local read "Magnification len live scar"() -> (w1322:string)
            n1264 = Not(x=w1311) -> (.not. x?=w1312:bool)
            n1265 = local write "Cap Live Image"(w1312) -> ()
            n1266 = case shown="\"ISO 12156\"" w1310 {
              tunnel: ["ASTM D6079" "ISO 12156"] -> w1309
              frame "ASTM D6079", Default {
              }
              frame "ISO 12156" {
              }
            }
            n1267 = case shown="\"5x\", Default" w1322 {
              tunnel: [w1325 w1326] -> w1321
              frame "5x", Default {
                n1268 = local read "5x Gain"() -> (w1325:dbl)
              }
              frame "10x" {
                # "5x"
                n1269 = local read "10x Gain"() -> (w1326:dbl)
              }
            }
            n1270 = local read "Image path"() -> (w1320:path)
            n1271 = local read "FILE 3"() -> (w1313:string)
            n1272 = call "EDGE DETCTION.vi"("GAIN VALUE"=w1321, "Image Path"=w1320) -> ("error out"=w1319:errorcluster, "return value"=w1318:cluster{string, string, dbl, dbl, dbl})  [unwired: 8 in]
            n1273 = Bundle By Name(cluster=T25 {"File Name"="", "Test Method"="", "Operator"="", "Fuel Description"="", "Date and time"=""} ("Main Ref"), "File Name"=w1313, "Test Method"=w1309) -> (w1314:T25)
            n1274 = call "duf file read.vi"("error in (no error)"=w1319, "Main Ref"=w1314) -> ("error out"=w1317:errorcluster, "Main Ref 2"=w1315:T25)  [unwired: 8 in]
            n1275 = call "EDGE DETECTION REPORT.vi"("error in (no error)"=w1317, "return value 2"=w1318, "Main Ref"=w1315) -> ()  [unwired: 8 in, 1 out]
          }
          frame #6 {
            n1276 = property on="Auto Scar Check  2" class="Clust (strict)"("Visible"=FALSE) -> ()  [unwired: 2 in, 2 out]
          }
          frame #7 {
            n1277 = call "CAMERA LIVE FEED FGV.vi"("Enum - Menu"=CAMERA_LIVE_FEED_ENUM."CAMERA MINIMIZE", "error in (no error)"=w1330) -> ()  [unwired: 8 in, 2 out]
            n1278 = local write "Main Dashboard Buttons"(T1."Home" ("Main Dashboard Buttons")) -> ()
            n1279 = local write "Main Tab"(T2."HOME" ("Main Tab")) -> ()
          }
        }
      }
    }
    n1280 = local read "Heater Button"() -> (w1183:bool)
    n1281 = case shown="True" w1185 {
      selector: w1185 -> [_ w1460]
      frame False {
      }
      frame True {
        n1282 = Not(x=w1460) -> (.not. x?=w1458:bool)
        n1283 = local write "Frequency"(w1458) -> ()
        n1284 = local write "Tab Control 2"(T6."Frequency" ("Tab Control 2")) -> ()
      }
    }
    n1285 = case shown="True" w1184 {
      selector: w1184 -> [_ w1457]
      frame False {
      }
      frame True {
        n1286 = Not(x=w1457) -> (.not. x?=w1455:bool)
        n1287 = local write "Air Temp vs Humidity"(w1455) -> ()
        n1288 = local write "Tab Control 2"(T6."Air Temp vs Rh" ("Tab Control 2")) -> ()
      }
    }
    n1289 = case shown="True" w1186 {
      selector: w1186 -> [_ w1463]
      frame False {
      }
      frame True {
        n1290 = Not(x=w1463) -> (.not. x?=w1461:bool)
        n1291 = local write "Sample Temperature"(w1461) -> ()
        n1292 = local write "Tab Control 2"(T6."Sample Temperature" ("Tab Control 2")) -> ()
      }
    }
    n1293 = case shown="\"Custom\"" w1182 {
      frame "ASTM D6079", Default {
        w1436 = "ASTM D6079 TEST CONDITIONS" ("Standard 2")
        n1294 = local write "Standard 2"(w1436) -> ()
        n1295 = local write "Standard"(w1436) -> ()
      }
      frame "ISO 12156" {
        w1437 = "ISO 12156 TEST CONDITIONS" ("Standard 2")
        n1296 = local write "Standard 2"(w1437) -> ()
        n1297 = local write "Standard"(w1437) -> ()
      }
      frame "CEC F-096-A-06" {
        w1438 = "CEC F-096-A-06 TEST CONDITIONS" ("Standard 2")
        n1298 = local write "Standard 2"(w1438) -> ()
        n1299 = local write "Standard"(w1438) -> ()
      }
      frame "Custom" {
        w1439 = "CUSTOM TEST CONDITIONS" ("Standard 2")
        n1300 = local write "Standard 2"(w1439) -> ()
        n1301 = local write "Standard"(w1439) -> ()
      }
    }
    n1302 = case shown="True" w1183 {
      frame False {
        n1303 = local write "Temperature On Command"(TRUE ("Temperature On Command")) -> ()
        n1304 = case shown="True" "Temperature Off Command" {
          selector: "Temperature Off Command" -> [_ w1443]
          frame False {
          }
          frame True {
            n1305 = Not(x=w1443) -> (.not. x?=w1442:bool)
            n1306 = local read "EVENT LOG"() -> (w1446:string)
            n1307 = local write "Temperature Off Command"(w1442) -> ()
            n1308 = call "Event Log.vi"("Content"="Heater Off", "EVENT LOG"=w1446) -> ("EVENT LOG"=w1445:string)  [unwired: 8 in, 1 out]
            n1309 = local write "EVENT LOG"(w1445) -> ()
          }
        }
      }
      frame True {
        n1310 = local write "Temperature Off Command"(TRUE ("Temperature Off Command")) -> ()
        n1311 = case shown="True" "Temperature On Command" {
          selector: "Temperature On Command" -> [_ w1450]
          frame False {
          }
          frame True {
            n1312 = Not(x=w1450) -> (.not. x?=w1449:bool)
            n1313 = local write "Temperature On Command"(w1449) -> ()
            n1314 = disable-structure shown="Enabled" {
              disable-tunnel: "Heater On" -> [w1452 _]
              frame Enabled {
                n1315 = local read "EVENT LOG"() -> (w1453:string)
                n1316 = call "Event Log.vi"("Content"=w1452, "EVENT LOG"=w1453) -> ("EVENT LOG"=w1454:string)  [unwired: 8 in, 1 out]
                n1317 = local write "EVENT LOG"(w1454) -> ()
              }
              frame Disabled {
              }
            }
          }
        }
      }
    }
    n1318 = local read "Main Tab"() -> (w1174:T2)
    n1319 = case shown="\"About\"" w1174 {
      frame "HOME", Default {
        w1217 = T19."Enabled" ("Disabled")
        n1320 = local read "Service Password enable"() -> (w1219:bool)
        n1321 = property on="Imaging" class="Bool (strict)"("DisabledEnum"=w1217) -> ()  [unwired: 2 in, 2 out]
        n1322 = property on="Dashboard" class="Bool (strict)"("DisabledEnum"=w1217) -> ()  [unwired: 2 in, 2 out]
        n1323 = property on="Test Setup" class="Bool (strict)"("DisabledEnum"=w1217) -> ()  [unwired: 2 in, 2 out]
        n1324 = property on="Analysis" class="Bool (strict)"("DisabledEnum"=w1217) -> ()  [unwired: 2 in, 2 out]
        n1325 = property on="Home" class="Bool (strict)"("DisabledEnum"=w1217) -> ()  [unwired: 2 in, 2 out]
        n1326 = property on="Report" class="Bool (strict)"("DisabledEnum"=w1217) -> ()  [unwired: 2 in, 2 out]
        n1327 = property on="Main Dashboard Buttons" class="RadioBtnsControl (strict)"("DisabledEnum"=w1217) -> ()  [unwired: 2 in, 2 out]
        n1328 = property on="Calibration" class="Bool (strict)"("DisabledEnum"=w1217) -> ()  [unwired: 2 in, 2 out]
        n1329 = case shown="True" w1219 {
          tunnel: [T19."Disabled" ("Disabled") T19."Enabled" ("Disabled")] -> w1218
          frame False {
          }
          frame True {
          }
        }
        n1330 = property on="About" class="Bool (strict)"("DisabledEnum"=w1218) -> ()  [unwired: 2 in, 2 out]
      }
      frame "Test Setup" {
        w1224 = T19."Enabled" ("Disabled")
        n1331 = local read "Service Password enable"() -> (w1223:bool)
        n1332 = property on="Dashboard" class="Bool (strict)"("DisabledEnum"=T19."Disabled" ("Disabled")) -> ()  [unwired: 2 in, 2 out]
        n1333 = property on="Imaging" class="Bool (strict)"("DisabledEnum"=w1224) -> ()  [unwired: 2 in, 2 out]
        n1334 = property on="Analysis" class="Bool (strict)"("DisabledEnum"=w1224) -> ()  [unwired: 2 in, 2 out]
        n1335 = property on="Home" class="Bool (strict)"("DisabledEnum"=w1224) -> ()  [unwired: 2 in, 2 out]
        n1336 = property on="Report" class="Bool (strict)"("DisabledEnum"=w1224) -> ()  [unwired: 2 in, 2 out]
        n1337 = property on="Test Setup" class="Bool (strict)"("DisabledEnum"=w1224) -> ()  [unwired: 2 in, 2 out]
        n1338 = case shown="True" w1223 {
          tunnel: [T19."Disabled" ("Disabled") T19."Enabled" ("Disabled")] -> w1222
          frame False {
          }
          frame True {
          }
        }
        n1339 = property on="About" class="Bool (strict)"("DisabledEnum"=w1222) -> ()  [unwired: 2 in, 2 out]
      }
      frame "Adv Scar" {
        w1231 = T19."Enabled" ("Disabled")
        n1340 = property on="Dashboard" class="Bool (strict)"("DisabledEnum"=T19."Disabled" ("Disabled")) -> ()  [unwired: 2 in, 2 out]
        n1341 = property on="Imaging" class="Bool (strict)"("DisabledEnum"=w1231) -> ()  [unwired: 2 in, 2 out]
        n1342 = property on="Analysis" class="Bool (strict)"("DisabledEnum"=w1231) -> ()  [unwired: 2 in, 2 out]
        n1343 = property on="Home" class="Bool (strict)"("DisabledEnum"=w1231) -> ()  [unwired: 2 in, 2 out]
        n1344 = property on="Report" class="Bool (strict)"("DisabledEnum"=w1231) -> ()  [unwired: 2 in, 2 out]
        n1345 = property on="Test Setup" class="Bool (strict)"("DisabledEnum"=w1231) -> ()  [unwired: 2 in, 2 out]
        n1346 = local read "Service Password enable"() -> (w1229:bool)
        n1347 = case shown="True" w1229 {
          tunnel: [T19."Disabled" ("Disabled") T19."Enabled" ("Disabled")] -> w1228
          frame False {
          }
          frame True {
          }
        }
        n1348 = property on="About" class="Bool (strict)"("DisabledEnum"=w1228) -> ()  [unwired: 2 in, 2 out]
      }
      frame "Calibration" {
        w1234 = T19."Enabled" ("Disabled")
        n1349 = property on="Dashboard" class="Bool (strict)"("DisabledEnum"=T19."Disabled" ("Disabled")) -> ()  [unwired: 2 in, 2 out]
        n1350 = property on="Imaging" class="Bool (strict)"("DisabledEnum"=w1234) -> ()  [unwired: 2 in, 2 out]
        n1351 = property on="Analysis" class="Bool (strict)"("DisabledEnum"=w1234) -> ()  [unwired: 2 in, 2 out]
        n1352 = property on="Home" class="Bool (strict)"("DisabledEnum"=w1234) -> ()  [unwired: 2 in, 2 out]
        n1353 = property on="Report" class="Bool (strict)"("DisabledEnum"=w1234) -> ()  [unwired: 2 in, 2 out]
        n1354 = property on="Test Setup" class="Bool (strict)"("DisabledEnum"=w1234) -> ()  [unwired: 2 in, 2 out]
        n1355 = local read "Service Password enable"() -> (w1236:bool)
        n1356 = property on="Calibration" class="Bool (strict)"("DisabledEnum"=w1234) -> ()  [unwired: 2 in, 2 out]
        n1357 = case shown="True" w1236 {
          tunnel: [T19."Disabled" ("Disabled") T19."Enabled" ("Disabled")] -> w1235
          frame False {
          }
          frame True {
          }
        }
        n1358 = property on="About" class="Bool (strict)"("DisabledEnum"=w1235) -> ()  [unwired: 2 in, 2 out]
      }
      frame "Adv Scar Report" {
        w1242 = T19."Enabled" ("Disabled")
        n1359 = property on="Dashboard" class="Bool (strict)"("DisabledEnum"=T19."Disabled" ("Disabled")) -> ()  [unwired: 2 in, 2 out]
        n1360 = property on="Imaging" class="Bool (strict)"("DisabledEnum"=w1242) -> ()  [unwired: 2 in, 2 out]
        n1361 = property on="Analysis" class="Bool (strict)"("DisabledEnum"=w1242) -> ()  [unwired: 2 in, 2 out]
        n1362 = property on="Home" class="Bool (strict)"("DisabledEnum"=w1242) -> ()  [unwired: 2 in, 2 out]
        n1363 = property on="Report" class="Bool (strict)"("DisabledEnum"=w1242) -> ()  [unwired: 2 in, 2 out]
        n1364 = property on="Test Setup" class="Bool (strict)"("DisabledEnum"=w1242) -> ()  [unwired: 2 in, 2 out]
        n1365 = local read "Service Password enable"() -> (w1241:bool)
        n1366 = case shown="True" w1241 {
          tunnel: [T19."Disabled" ("Disabled") T19."Enabled" ("Disabled")] -> w1240
          frame False {
          }
          frame True {
          }
        }
        n1367 = property on="About" class="Bool (strict)"("DisabledEnum"=w1240) -> ()  [unwired: 2 in, 2 out]
      }
      frame "Compare Files" {
        w1248 = T19."Enabled" ("Disabled")
        n1368 = local read "Service Password enable"() -> (w1247:bool)
        n1369 = property on="Dashboard" class="Bool (strict)"("DisabledEnum"=T19."Disabled" ("Disabled")) -> ()  [unwired: 2 in, 2 out]
        n1370 = property on="Imaging" class="Bool (strict)"("DisabledEnum"=w1248) -> ()  [unwired: 2 in, 2 out]
        n1371 = property on="Analysis" class="Bool (strict)"("DisabledEnum"=w1248) -> ()  [unwired: 2 in, 2 out]
        n1372 = property on="Home" class="Bool (strict)"("DisabledEnum"=w1248) -> ()  [unwired: 2 in, 2 out]
        n1373 = property on="Report" class="Bool (strict)"("DisabledEnum"=w1248) -> ()  [unwired: 2 in, 2 out]
        n1374 = property on="Test Setup" class="Bool (strict)"("DisabledEnum"=w1248) -> ()  [unwired: 2 in, 2 out]
        n1375 = case shown="True" w1247 {
          tunnel: [T19."Disabled" ("Disabled") T19."Enabled" ("Disabled")] -> w1246
          frame False {
          }
          frame True {
          }
        }
        n1376 = property on="About" class="Bool (strict)"("DisabledEnum"=w1246) -> ()  [unwired: 2 in, 2 out]
      }
      frame "Acquire" {
        n1377 = local read "Service Password enable"() -> (w1253:bool)
        n1378 = property on="Test Setup" class="Bool (strict)"("DisabledEnum"=T19."Disabled" ("Disabled")) -> ()  [unwired: 2 in, 2 out]
        n1379 = local read "Auto Start Test"() -> (w1255:bool)
        n1380 = local read "RUN"() -> (w1257:bool)
        n1381 = case shown="True" w1253 {
          tunnel: [T19."Disabled" ("Disabled") T19."Enabled" ("Disabled")] -> w1254
          frame False {
          }
          frame True {
          }
        }
        n1382 = Or(x=w1257, y=w1255) -> (x .or. y?=w1256:bool)
        n1383 = case shown="True" w1256 {
          tunnel: [T19."Enabled" ("Disabled") T19."Disabled" ("Disabled")] -> w1252
          frame False {
          }
          frame True {
          }
        }
        n1384 = property on="About" class="Bool (strict)"("DisabledEnum"=w1254) -> ()  [unwired: 2 in, 2 out]
        n1385 = property on="Imaging" class="Bool (strict)"("DisabledEnum"=w1252) -> ()  [unwired: 2 in, 2 out]
        n1386 = property on="Dashboard" class="Bool (strict)"("DisabledEnum"=w1252) -> ()  [unwired: 2 in, 2 out]
        n1387 = property on="Analysis" class="Bool (strict)"("DisabledEnum"=w1252) -> ()  [unwired: 2 in, 2 out]
        n1388 = property on="Home" class="Bool (strict)"("DisabledEnum"=w1252) -> ()  [unwired: 2 in, 2 out]
        n1389 = property on="Report" class="Bool (strict)"("DisabledEnum"=w1252) -> ()  [unwired: 2 in, 2 out]
        n1390 = property on="Calibration" class="Bool (strict)"("DisabledEnum"=w1252) -> ()  [unwired: 2 in, 2 out]
      }
      frame "About" {
        n1391 = local read "FILE"() -> (w1271:string)
        n1392 = local read "TEST FILE NAM,E SAVED"() -> (w1264:bool)
        n1393 = call <vilib>:"Trim Whitespace.vi"("string"=w1271) -> ("trimmed string"=w1270:string)  [unwired: 1 in]
        n1394 = local read "Auto Start Test"() -> (w1274:bool)
        n1395 = String Length(string=w1270) -> (length=w1269:i32)
        n1396 = Greater?(x=w1269, y=1) -> (0:w1266:bool)
        n1397 = And(x=w1266, y=w1264) -> (x .and. y?=w1265:bool)
        n1398 = local read "RUN"() -> (w1276:bool)
        n1399 = case shown="True" w1265 {
          tunnel: [T19."Disabled" ("Disabled") T19."Enabled" ("Disabled")] -> w1267
          frame False {
          }
          frame True {
          }
        }
        n1400 = Or(x=w1276, y=w1274) -> (x .or. y?=w1275:bool)
        n1401 = property on="About" class="Bool (strict)"("DisabledEnum"=T19."Enabled" ("Disabled")) -> ()  [unwired: 2 in, 2 out]
        n1402 = case shown="False" w1275 {
          tunnel: [T19."Enabled" ("Disabled") T19."Disabled" ("Disabled")] -> w1273
          frame False {
          }
          frame True {
          }
        }
        n1403 = property on="Dashboard" class="Bool (strict)"("DisabledEnum"=w1267) -> ()  [unwired: 2 in, 2 out]
        n1404 = property on="Test Setup" class="Bool (strict)"("DisabledEnum"=T19."Disabled" ("Disabled")) -> ()  [unwired: 2 in, 2 out]
        n1405 = property on="Imaging" class="Bool (strict)"("DisabledEnum"=w1273) -> ()  [unwired: 2 in, 2 out]
        n1406 = property on="Analysis" class="Bool (strict)"("DisabledEnum"=w1273) -> ()  [unwired: 2 in, 2 out]
        n1407 = property on="Home" class="Bool (strict)"("DisabledEnum"=w1273) -> ()  [unwired: 2 in, 2 out]
        n1408 = property on="Report" class="Bool (strict)"("DisabledEnum"=w1273) -> ()  [unwired: 2 in, 2 out]
      }
    }
    n1409 = local read "Quit"() -> (w1201:bool)
    "Single" <- "Single - Graph"
  }
  n1410 = disable-structure shown="Disabled" {
    disable-tunnel: [w1553 _] -> w40
    disable-tunnel: _ -> [w1552 _]
    frame Disabled {
      n1411 = while {
        tunnel: w1552 -> [_]
        tunnel: [w1554] -> w1553
        tunnel: [w1555] -> _
        i -> [w1555]
        stop <- w1554 stop-if-true
        w1571 = u16 10 items=["1.0"=10, "1.5"=15, "2.0"=20] ("stop bits (10: 1 bit)")
        n1412 = Wait (ms)(milliseconds to wait=u32 10) -> ()  [unwired: 1 out]
        n1413 = call-poly "VISA Configure Serial Port"("VISA resource name"=refnum<visa-resource-name> "ASRL1::INSTR" ("COM PORT"), "timeout (10sec)"=u32 10, "baud rate (9600)"=u32 57600, "data bits (8)"=u16 8, "stop bits (10: 1 bit)"=w1571) -> ("VISA resource name out"=w1557:refnum<visa-resource-name>, "error out"=w1566:errorcluster)  [unwired: 9 in]
        n1414 = VISA Read(VISA resource name=w1557, byte count=u32 2 ("byte count (0)")) -> (read buffer=w1565:string)  [unwired: 1 in, 3 out]
        n1415 = String Subset(string=w1565, offset (0)=0, length (rest)=2 ("length (rest)")) -> (substring=w1564:string)
        n1416 = Match Pattern(string=w1564, regular expression="<>") -> (offset past match=w1561:i32)  [unwired: 1 in, 3 out]
        n1417 = Greater Or Equal?(x=w1561, y=0) -> (x >= y?=w1556:bool)
        n1418 = case shown="True" w1556 {
          tunnel: w1557 -> [_ w1575]
          tunnel: w1566 -> [_ w1574]
          frame False {
          }
          frame True {
            n1419 = VISA Read(VISA resource name=w1575, byte count=u32 32 ("byte count (0)"), error in (no error)=w1574) -> (read buffer=w1573:string)  [unwired: 3 out]
            n1420 = String Subset(string=w1573, offset (0)=0, length (rest)=8 ("length (rest)")) -> (substring=w1577:string)
            n1421 = String Subset(string=w1573, offset (0)=8, length (rest)=8 ("length (rest)")) -> (substring=w1578:string)
            n1422 = Decimal String To Number(string=w1578) -> (number=w1585:i32)  [unwired: 2 in, 1 out]
            n1423 = Decimal String To Number(string=w1577) -> (number=w1581:i32)  [unwired: 2 in, 1 out]
            n1424 = Divide(x=w1585, y=10000) -> ()  [unwired: 1 out]
            n1425 = Divide(x=w1581, y=1000000) -> ()  [unwired: 1 out]
          }
        }
        n1426 = local read "Quit"() -> (w1554:bool)
      }
    }
    frame Enabled {
    }
  }
  n1427 = while {
    stop <- w1589 stop-if-true
    n1428 = local read "error out 11"() -> (w1587:errorcluster)
    n1429 = case shown="No Error" w1587 {
      frame No Error {
        n1430 = local read "UNI READ"() -> (w1596:string)
        n1431 = String To Byte Array(string=w1596) -> (unsigned byte array=w1595:u8[])
        n1432 = Array Size(array=w1595) -> (size(s)=w1594:i32)
        n1433 = formula code="// 1. Declare ALL internal variables at the very top (using 'int' and 'float')\nint i = 0;\nint k = 0;\nint start_idx = -1;\nint end_idx = -1;\nint phase = 0;\nint sign0 = 1;\nint sign1 = 1;\nint ch0_val = 0;   \nint ch1_val = 0;   \nfloat ch0_raw = 0.0;\nfloat ch1_raw = 0.0;\n\n// Initialize tracking variables using 'float'\nfloat max_ch0 = -9999999.0;\nfloat min_ch0 =  9999999.0;\nfloat max_ch1 = -9999999.0;\nfloat min_ch1 =  9999999.0;\n\n// Default outputs to 0\nvalid_data = 0;\nLVDT_Min_V = 0.0; LVDT_Max_V = 0.0; LVDT_P2P_V = 0.0;\nPiezo_P2P = 0.0; Friction_N = 0.0; COF = 0.0;\n\n// Scan the byte array for packets\nfor (i = 0; i < array_size - 1; i++) {\n    // Look for the start delimiter '*' (ASCII 42)\n    if (raw_bytes[i] == 42) {\n        start_idx = i;\n    }\n    \n    // Look for the end delimiter ';&' (ASCII 59 and 38)\n    if (raw_bytes[i] == 59 && raw_bytes[i+1] == 38 && start_idx != -1) {\n        end_idx = i;\n        ch0_val = 0;\n        ch1_val = 0;\n        sign0 = 1;\n        sign1 = 1;\n        phase = 0; // 0 = parsing Ch0, 1 = parsing Ch1\n\n        // Parse ASCII characters inside this specific packet frame\n        for (k = start_idx + 1; k < end_idx; k++) {\n            if (raw_bytes[k] == 45) { // Negative sign '-'\n                if (phase == 0) sign0 = -1;\n                else sign1 = -1;\n            }\n            else if (raw_bytes[k] == 59) { // Separator ';'\n                phase = 1; \n            }\n            else if (raw_bytes[k] >= 48 && raw_bytes[k] <= 57) { // Numbers '0'-'9'\n                if (phase == 0) {\n                    ch0_val = (ch0_val * 10) + (raw_bytes[k] - 48);\n                } else {\n                    ch1_val = (ch1_val * 10) + (raw_bytes[k] - 48);\n                }\n            }\n        }\n\n        // FIXED: Removed the C-style (float) cast syntax. LabVIEW auto-promotes this seamlessly.\n        ch0_raw = ch0_val * sign0;\n        ch1_raw = ch1_val * sign1;\n        valid_data = 1;\n\n        // Track Min/Max values across the entire chunk of frames\n        if (ch0_raw > max_ch0) max_ch0 = ch0_raw;\n        if (ch0_raw < min_ch0) min_ch0 = ch0_raw;\n        if (ch1_raw > max_ch1) max_ch1 = ch1_raw;\n        if (ch1_raw < min_ch1) min_ch1 = ch1_raw;\n\n        // Reset start_idx to find the next packet in the loop\n        start_idx = -1; \n    }\n}\n\n// Step 2: If valid packets were parsed, calculate physical metrics using user entries\nif (valid_data == 1) {\n    // LVDT Scaling\n    LVDT_Min_V = (min_ch0 * VREF) / ADC_Resolution;\n    LVDT_Max_V = (max_ch0 * VREF) / ADC_Resolution;\n    LVDT_P2P_V = LVDT_Max_V - LVDT_Min_V;\n\n    // Piezo, Friction & COF Scaling\n    Piezo_P2P = max_ch1 - min_ch1;\n    Friction_N = Piezo_P2P * PIEZO_CAL_FACTOR;\n    COF = Friction_N / NORMAL_FORCE;\n}"("raw_bytes"=w1595, "array_size"=w1594, "VREF"="VREF", "ADC_Resolution"="ADC_Resolution", "PIEZO_CAL_FACTOR"="PIEZO_CAL_FACTOR", "NORMAL_FORCE"="NORMAL_FORCE") -> ("valid_data"=→"Valid_data":dbl, "LVDT_Min_V"=→"LVDT MIN":dbl, "LVDT_Max_V"=→"LVDT MAX":dbl, "LVDT_P2P_V"=→"LVDT Peak":dbl, "Piezo_P2P"=→"pizo raw":dbl, "Friction_N"=→"Friction":dbl, "COF"=→"cof":dbl)
      }
      frame Error {
      }
    }
    n1434 = Wait (ms)(milliseconds to wait=u32 40) -> ()  [unwired: 1 out]
    n1435 = local read "Quit"() -> (w1589:bool)
  }
  n1436 = while {
    shift-right: [w1617] -> w53
    shift-left: _ -> [w1608]
    shift-right: [w1616] -> w52
    shift-left: errorcluster {"status"=TRUE, "code"=0, "source"="Init"} ("error IO") -> [w1610]
    tunnel: [w1605] -> w43
    tunnel: [w1615] -> _
    i -> [w1615]
    stop <- w1605 stop-if-true
    n1437 = local read "Port 1a"() -> (w1611:bool)
    n1438 = local read "Port 3"() -> (w1612:bool)
    n1439 = local read "Com Port 1"() -> (w1609:refnum<visa-resource-name>)
    n1440 = Or(x=w1612, y=w1611) -> (x .or. y?=w1614:bool)
    n1441 = Unbundle(w1610) -> ("status"=→"Port 3":bool)  [unwired: 2 out]
    n1442 = Not Equal?(x=w1609, y=w1608) -> (x != y?=w1606:bool)
    n1443 = case shown="True" w1614 {
      frame False {
        w1620 = TRUE ("Visible")
        n1444 = property on="Port 1a" class="Bool (strict)"("Visible"=w1620) -> ()  [unwired: 2 in, 2 out]
        n1445 = property on="Port 3" class="Bool (strict)"("Visible"=w1620) -> ()  [unwired: 2 in, 2 out]
      }
      frame True {
        w1621 = TRUE ("Visible")
        n1446 = property on="Port 1a" class="Bool (strict)"("Visible"=w1621) -> ()  [unwired: 2 in, 2 out]
        n1447 = property on="Port 3" class="Bool (strict)"("Visible"=w1621) -> ()  [unwired: 2 in, 2 out]
      }
    }
    n1448 = Wait (ms)(milliseconds to wait=u32 40) -> ()  [unwired: 1 out]
    n1449 = case shown="True" w1606 {
      tunnel: [w1618 errorcluster {"status"=TRUE, "code"=0, "source"="Init"} ("error out")] -> w1607
      tunnel: w1610 -> [w1618 _]
      frame False {
      }
      frame True {
      }
    }
    "error out 11" <- w1607
    n1450 = case shown="No Error" w1607 {
      selector: w1607 -> [w1628 w1646]
      tunnel: [w1631 w1650] -> w1617
      tunnel: [w1630 w1644] -> w1616
      tunnel: w1608 -> [w1629 w1648]
      frame No Error {
        n1451 = property class="Instr"(reference=w1629, error in=w1628) -> (reference out=w1626:refnum<visa-resource-name>, error out=w1627:errorcluster, "Serial Settings:Number of Bytes at Serial Port"=w1623:u32)
        n1452 = Greater?(x=w1623, y=u32 5) -> (0:w1622:bool)
        n1453 = Not(x=w1622) -> (.not. x?=→"Port 1a":bool)
        n1454 = while {
